vi "Stop Core.vi"(10 "final error code":i32, 11 "Command in":refnum<class "Command State Actor.lvclass">) -> (3 "Command out":refnum<class "Command State Actor.lvclass">)   [LabVIEW 2013, in "Command State Actor.lvlib" / "Command State Actor.lvclass"]
doc: "(<B>Filename</B>: Actor Framework.lvlib:Actor.lvclass:Stop Core.vi)\n\nDefines what the actor does before it stops. Use the <B>final error code</B> input to determine whether the actor shut down in response to an error.\n\nBy default, this method does nothing. A descendant class may override it to define behavior, such as shutting down any processes the actor initiated in its override of the Actor Core method."
uses:
  Command State Actor.lvclass
  <vilib>/ni/Actors/State Actor/State Actor/State Actor.lvclass
  Command State Actor.lvclass/Command State Actor.ctl
  <vilib>/ActorFramework/Stop Msg/Stop Msg.lvclass/Stop Msg.ctl
  <vilib>/ActorFramework/Message Enqueuer/Message Enqueuer.lvclass/Message Enqueuer.ctl
  <vilib>/ActorFramework/Stop Msg/Send Emergency Stop.vi
  <vilib>/ActorFramework/Stop Msg/Send Normal Stop.vi
  <vilib>/ActorFramework/Message Enqueuer/Enqueue Critical.vi
  <vilib>/ActorFramework/Message Enqueuer/Enqueue.vi
  <vilib>/ActorFramework/Message Priority Queue/Priority Enqueue.vi
  <vilib>/ActorFramework/Stop Msg/Stop Msg.lvclass
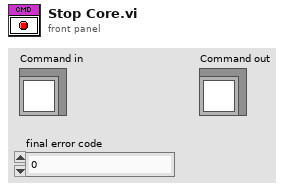
[diagram p1: front panel]
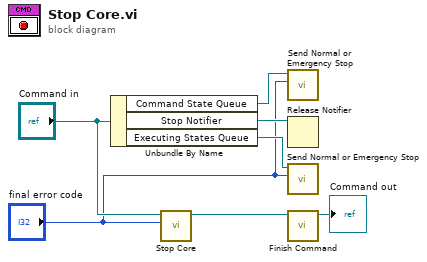
[diagram p0: block diagram]
diagram:
  n1 = Unbundle By Name("Command in") -> ("Command State Queue"=w3:refnum<class "Message Enqueuer.lvclass">, "Stop Notifier"=w4:refnum<notifier>, "Executing States Queue"=w2:refnum<class "Message Enqueuer.lvclass">)
  n2 = call-parent "Stop Core.vi"("final error code"="final error code", "Actor in"="Command in") -> ("Actor out"=w7:refnum<class "Command State Actor.lvclass">)  [unwired: 9 in]
  n3 = call <vilib>:"Send Normal or Emergency Stop.vi"("final error code"="final error code", "Message Enqueuer"=w3) -> ()  [unwired: 9 in, 1 out]
  n4 = Release Notifier(notifier=w4) -> ()  [unwired: 2 in, 3 out]
  n5 = call <vilib>:"Send Normal or Emergency Stop.vi"("final error code"="final error code", "Message Enqueuer"=w2) -> ()  [unwired: 9 in, 1 out]
  n6 = call-dynamic "Finish Command.vi"("Command in"=w7) -> ("Command out"=→"Command out":refnum<class "Command State Actor.lvclass">)  [unwired: 9 in, 1 out]
